vi "myRIO_BRig_RT_dataExp_Tcycle_Cue1Penalty_Audio.vi"() -> (2 "output_Tcycle_Cue1Penalty_Audio":i32)   [LabVIEW 2014]
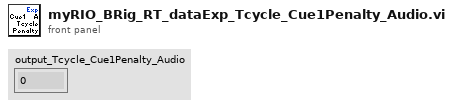
[diagram p1: front panel]
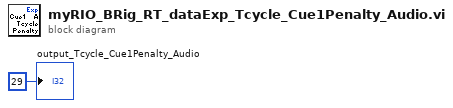
[diagram p0: block diagram]
diagram:
  "output_Tcycle_Cue1Penalty_Audio" <- 29 ("output_iBlock")
